vi "Measurement UI well fit.vi"() -> ()   [LabVIEW 2025, in "auto-vision-plugin UI.lvlib"]
uses:
  auto-vision-plugin UI.lvlib
  <vilib>/userDefined/Silver/nirio_resource_slv.ctl
panel:
  out "FRAME COUNT":u64
  in  "IMAGE SAVE FORMAT":enum32{"Item 0", "Item 1"}(radio)
  out "IMAGE DATA":string="IMAGE RESOLUTION: 800x600 - RAW12"
  in  "PAUSE":bool
  in  "CAPTURE":bool
  in  "PATH TO IMAGE CAPTURE":path=path "C:/dev/examplePLUGIN/1487 HIHO GSE/scripts/TDMS"
  in  "INTERPRETATION":u16(ring) items=["Grayscale", "Bayer", "RGB", "YUV422", "YUV420", "Legacy YUV420"]
  in  "PATTERN":u16(ring) items=["GB", "GR", "BG", "RG"]
  in  "ALGORITHM":u16(ring) items=["BILINEAR", "VNG"]
  in  "BLUE GAIN":dbl
  in  "GREEN GAIN":dbl
  in  "RED GAIN":dbl
  in  "PIXEL SKIP COUNT":u16
  in  "LINE SKIP COUNT":u16
  in  "FRAME SKIP COUNT":u16
  in  "VIRTUAL CHANNEL":u16
  in  "PAYLOAD DATA TYPE":T1(ring)=enum."RAW 12"
  in  "SERIAL (SI) CHANNEL":string="SI0"
  out "SOURCE RATE (fps)":u64
  in  "SERIAL INPUT ACTIVE LANE COUNT":u16(ring) items=["1 LANE"=1, "2 LANE"=2, "4 LANE"=4]
  in  "REF. CLK FREQUENCY (Hz)":dbl
  in  "POWER OVER COAX (POC) SOURCE":u16(ring) items=["NONE", "INTERNAL", "AUXILIARY"]
  out "STATE MESSAGE":string
  out "ERROR":bool
  in  "CSI-2 DATA SOURCE":u16(ring) items=["CORRECTED", "RAW"]
  in  "PATH TO CONFIGURATION SCRIPT":path=path "C:/dev/examplePLUGIN/1487 HIHO GSE/scripts/Image Receiver Scripts/9296A_RAW8.cpp"
  out "POC CURRENT (A)":u64
  out "POC VOLTAGE (V)":u64
  out "ACQ. DURATION (s)":u64
  out "ACQ. IN PROGRESS":bool
  in  "LOGGED PACKETS":u64
  in  "LOG PACKETS TO DISK":bool
  in  "RIO DEVICE":T2
  out "DISPLAY":T3(plugin-control)
  # "FPGA DISPLAY PARAMETER"
  # "TDMS dir - will be labview defautl \nbitfile - will be chonse based on devicve type"
  # "RAW DISPLAY PARAMETERS"
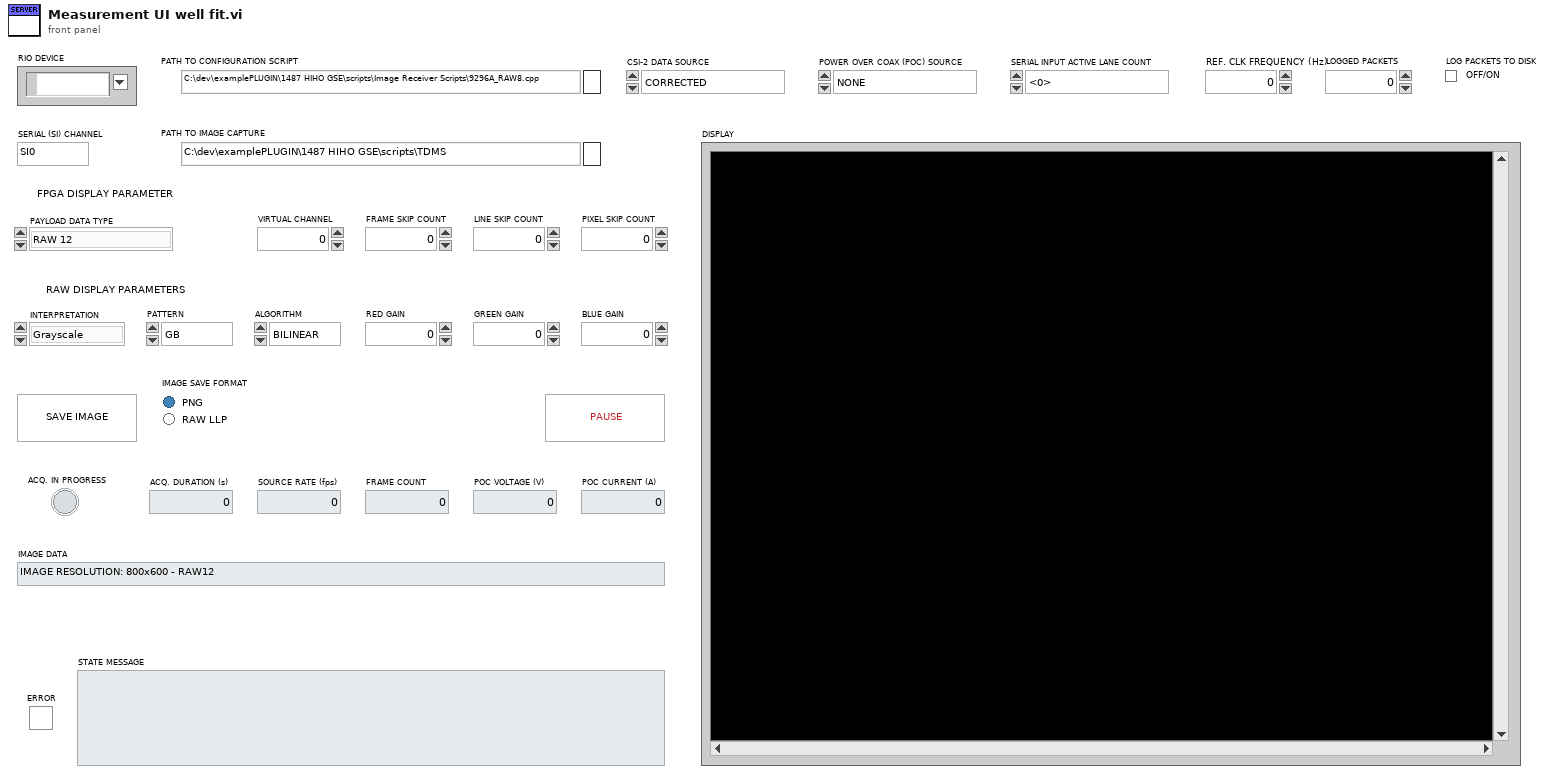
[diagram p1: front panel]
types:
  T1 = enum8{"Frame Start", "Frame End", "Line Start", "Line End", "End of Transmission", "Reserved 0", "Reserved 1", "Reserved 2", "Generic Short Packet 1", "Generic Short Packet 2", "Generic Short Packet 3", "Generic Short Packet 4", "Generic Short Packet 5", "Generic Short Packet 6", "Generic Short Packet 7", "Generic Short Packet 8", "Null", "Blanking Data", "Embedded 8-bit non Image Data", "Generic Long Packet 1", "Generic Long Packet 2", "Generic Long Packet 3", "Generic Long Packet 4", "Reserved 3", "YUV420 8-bit", "YUV420 10-bit", "Legacy YUV420 8-bit", "Reserved 4", "YUV420 8-bit Chroma Shifted", "YUV420 10-bit Chroma Shifted", "YUV422 8-bit", "YUV422 10-bit", "RGB444", "RGB555", "RGB565", "RGB666", "RGB888", "Reserved 5", "Reserved 6", "RAW 24", "RAW 6", "RAW 7", "RAW 8", "RAW 10", "RAW 12", "RAW 14", "RAW 16", "RAW 20", "User Defined 8-bit Data 1", "User Defined 8-bit Data 2", "User Defined 8-bit Data 3", "User Defined 8-bit Data 4", "User Defined 8-bit Data 5", "User Defined 8-bit Data 6", "User Defined 8-bit Data 7", "User Defined 8-bit Data 8", "USL Command", "Reserved 7", "Reserved 8", "Reserved 9", "Reserved 10", "Reserved 11", "Reserved 12", "LRTE EPD Spacer"}
  T2 = typedef "nirio_resource_slv.ctl" = tag
  T3 = typedef "IMAQ Image.ctl" = refnum<image>
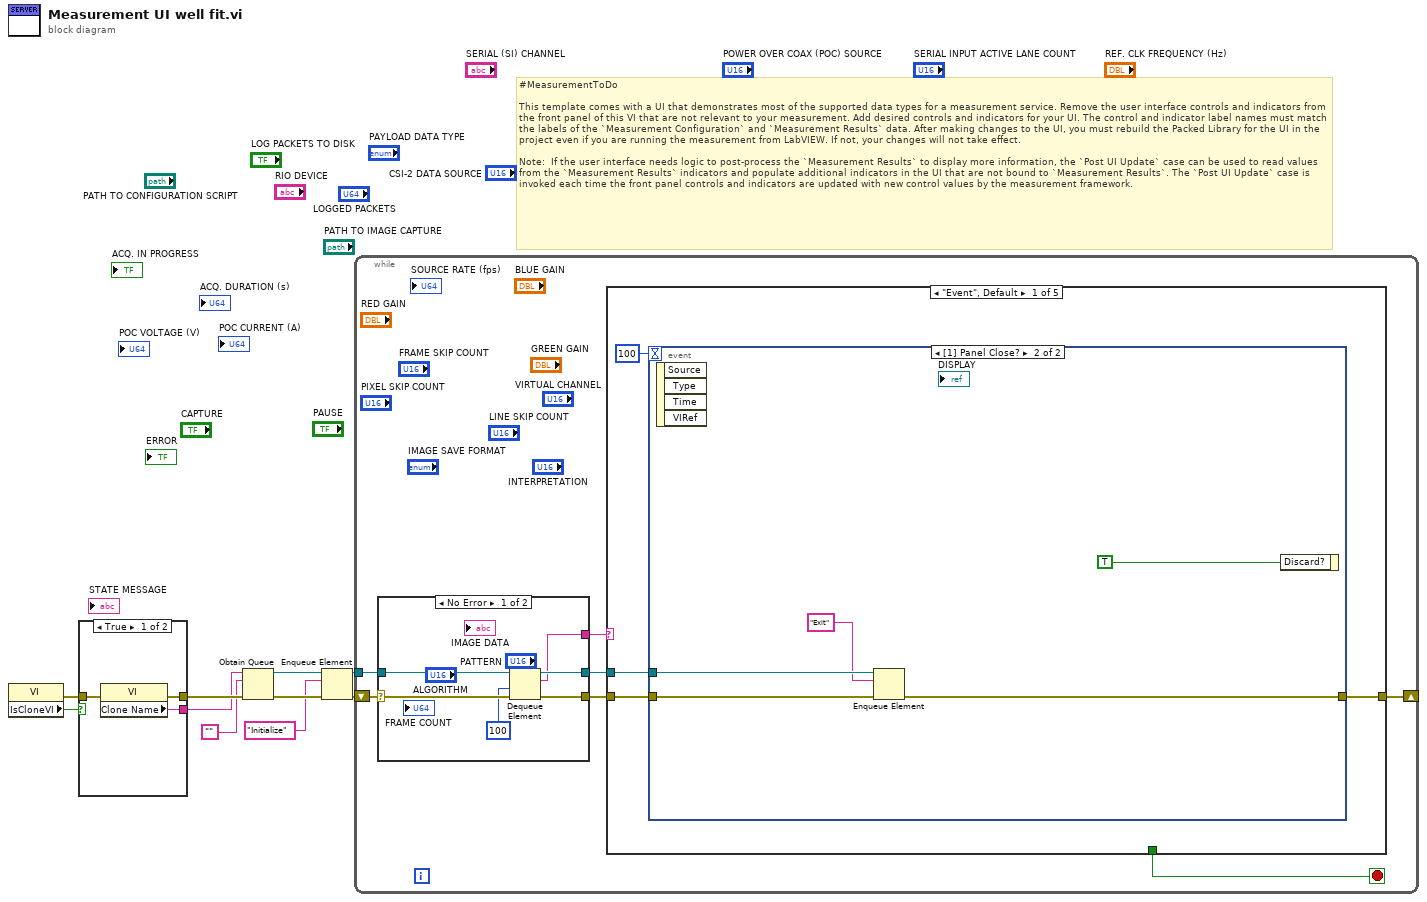
[diagram p0: block diagram]
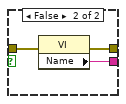
[diagram p2: hidden frame]
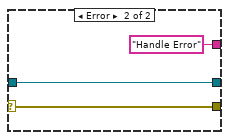
[diagram p3: hidden frame]
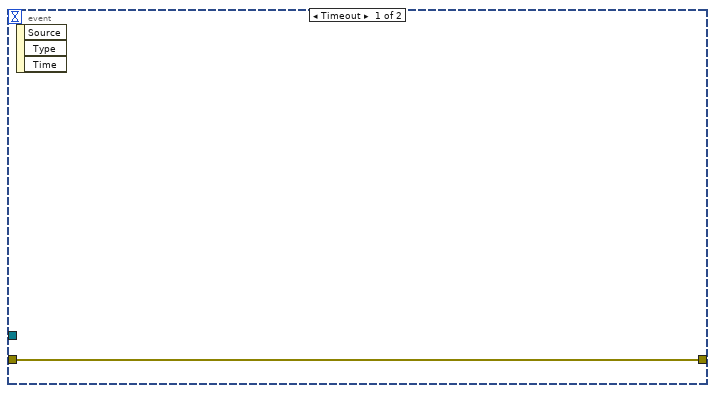
[diagram p4: hidden frame]
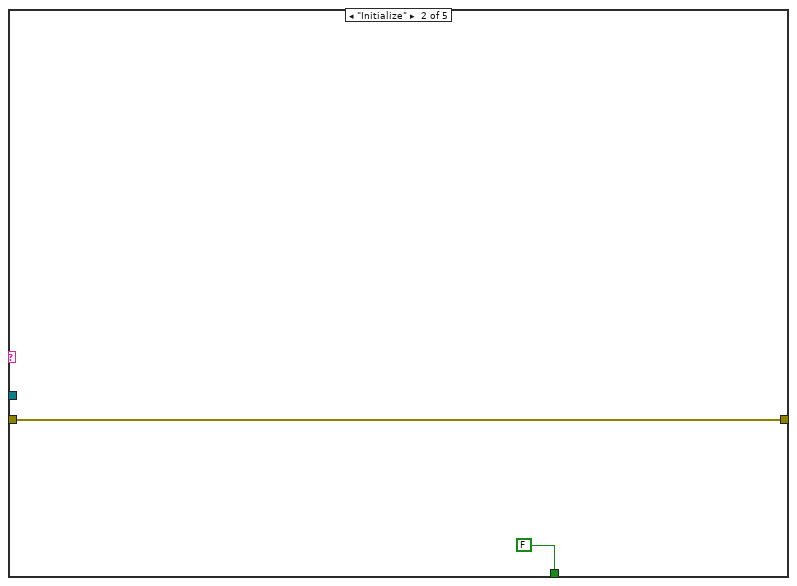
[diagram p5: hidden frame]
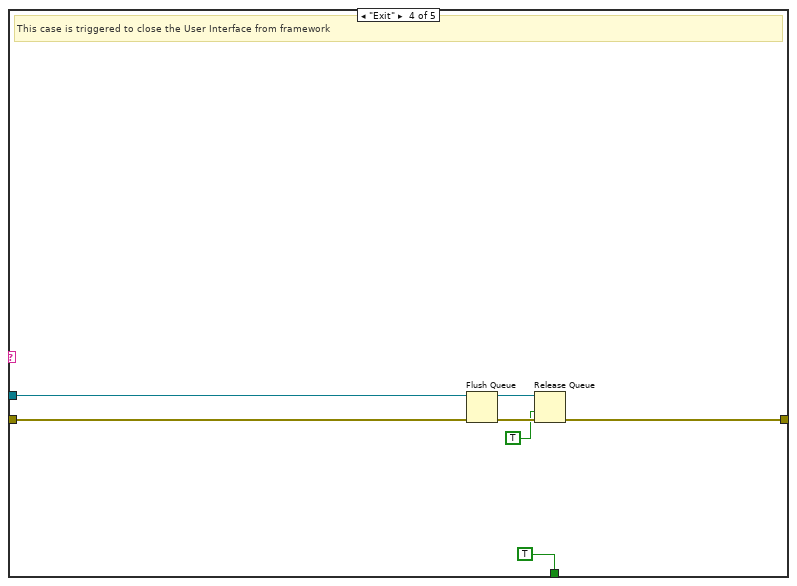
[diagram p7: hidden frame]
diagram:
  # "#MeasurementToDo  \n\nThis template comes with a UI that demonstrates most of the supported data types for a measurement service. Remove the user interface controls and indicators from the front panel of this VI that are not relevant to your measurement. Add desired controls and indicators for your UI. The control and indicator label names must match the labels of the `Measurement Configuration` and `Measurement Results` data. After making changes to the UI, you must rebuild the Packed Library for the UI in the project even if you are running the measurement from LabVIEW. If not, your changes will not take effect.\n\nNote:  If the user interface needs logic to post-process the `Measurement Results` to display more information, the `Post UI Update` case can be used to read values from the `Measurement Results` indicators and populate additional indicators in the UI that are not bound to `Measurement Results`. The `Post UI Update` case is invoked each time the front panel controls and indicators are updated with new control values by the measurement framework."
  n1 = property class="VI"() -> (error out=w1:errorcluster, "IsCloneVI"=w2:bool)  [unwired: 2 in, 1 out]
  n2 = case shown="True" w2 {
    tunnel: [w13 w16] -> w10
    tunnel: [w12 w15] -> w9
    tunnel: w1 -> [w11 w14]
    frame True {
      n3 = property class="VI"(error in=w11) -> (error out=w13:errorcluster, "Clone Name"=w12:string)  [unwired: 1 in, 1 out]
    }
    frame False {
      n4 = property class="VI"(error in=w14) -> (error out=w16:errorcluster, "Name"=w15:string)  [unwired: 1 in, 1 out]
    }
  }
  n5 = Obtain Queue(name (unnamed)=w9, element data type="", error in (no error)=w10) -> (queue out=w6:refnum<queue>, error out=w8:errorcluster)  [unwired: 2 in, 1 out]
  n6 = Enqueue Element(queue=w6, element="Initialize", error in (no error)=w8) -> (queue out=w5:refnum<queue>, error out=w7:errorcluster)  [unwired: 1 in, 1 out]
  n7 = while {
    shift-right: [w18] -> _
    shift-left: w7 -> [w23]
    tunnel: w5 -> [w21]
    stop <- w17 stop-if-true
    n8 = case shown="No Error" w23 {
      selector: w23 -> [w29 w32]
      tunnel: [w28 w32] -> w22
      tunnel: w21 -> [w27 w31]
      tunnel: [w26 w31] -> w20
      tunnel: [w25 "Handle Error"] -> w19
      frame No Error {
        n9 = Dequeue Element(queue=w27, timeout in ms (-1)=100, error in (no error)=w29) -> (queue out=w26:refnum<queue>, element=w25:string, error out=w28:errorcluster)  [unwired: 1 out]
      }
      frame Error {
      }
    }
    n10 = case shown="\"Event\", Default" w19 {
      tunnel: w22 -> [w35 w44 w45 w52 w53]
      tunnel: w20 -> [w33 _ _ w50 _]
      tunnel: [w36 w44 w45 w47 w53] -> w18
      tunnel: [_ FALSE _ TRUE _] -> w17
      frame "Event", Default {
        n11 = event shown="[1] Panel Close?" {
          selector: _ -> [_ _]
          dyn-events: _ -> [_ _]
          timeout: 100 -> [_ _]
          tunnel: [w37 w40] -> w36
          tunnel: w35 -> [w37 w41]
          tunnel: w33 -> [_ w39]
          event Timeout {
            n12 = event-data() -> ()  [unwired: 1 in, 3 out]
          }
          event Panel Close? {
            n13 = event-data() -> ()  [unwired: 1 in, 4 out]
            n14 = Enqueue Element(queue=w39, element="Exit", error in (no error)=w41) -> (error out=w40:errorcluster)  [unwired: 1 in, 2 out]
            n15 = event-data("Discard?"=TRUE) -> ()  [unwired: 1 in, 1 out]
          }
        }
      }
      frame "Initialize" {
      }
      frame "Post UI Update" {
        # "This case will be triggered, after framework updates the User interface with result values."
      }
      frame "Exit" {
        # "This case is triggered to close the User Interface from framework"
        n16 = Flush Queue(queue=w50, error in (no error)=w52) -> (queue out=w49:refnum<queue>, error out=w48:errorcluster)  [unwired: 1 out]
        n17 = Release Queue(queue=w49, force destroy? (F)=TRUE, error in (no error)=w48) -> (error out=w47:errorcluster)  [unwired: 2 out]
      }
      frame "Handle Error" {
      }
    }
  }
